vi "Step Update Output.vi"(8 "error in (no error)":errorcluster, 10 "Output in":T1, 11 "Step in":refnum<class "Step.lvclass">) -> (0 "error out":errorcluster, 3 "Step out":refnum<class "Step.lvclass">)   [LabVIEW 2015, in "OutputUI.lvclass"]
uses:
  OutputUI.lvclass
  Step.lvclass
  Step/STEP_OUTPUT.ctl
  Step/OUTPUT_DATA_TYPE.ctl
  OUTPUT_CHECK_TYPE.ctl
  Step/OUTPUT_VALUE_TYPE.ctl
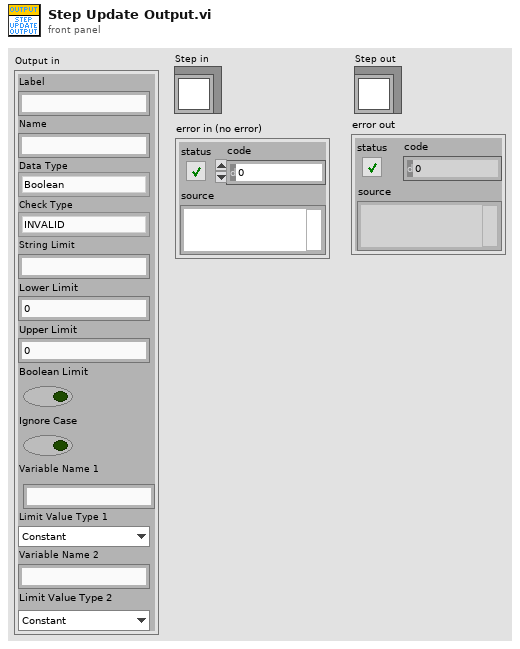
[diagram p1: front panel]
types:
  T1 = typedef "Step.lvclass/STEP_OUTPUT.ctl" = cluster{"Label":string, "Name":string, "Data Type":T2, "Check Type":T3, "String Limit":string, "Lower Limit":dbl, "Upper Limit":dbl, "Boolean Limit":bool, "Ignore Case":bool, "Variable Name 1":string, "Limit Value Type 1":T4, "Variable Name 2":string, "Limit Value Type 2":T4}
  T2 = typedef "Step.lvclass/OUTPUT_DATA_TYPE.ctl" = enum16{"Boolean", "String", "Numeric", "Other"}
  T3 = typedef "Step.lvclass/OUTPUT_CHECK_TYPE.ctl" = enum16{"INVALID", "DO_NOT_CHECK", "RECORD", "VARIABLE", "EQUAL", "NOT_EQUAL", "STR_CONTAINS", "STR_START_WITH", "STR_END_WITH", "STR_REGEX_MATCH", "NUM_GT", "NUM_LT", "NUM_GE", "NUM_LE", "NUM_RANGE", "NUM_RANGE_BDY"}
  T4 = typedef "Step.lvclass/OUTPUT_VALUE_TYPE.ctl" = enum16{"Constant", "Variable"}
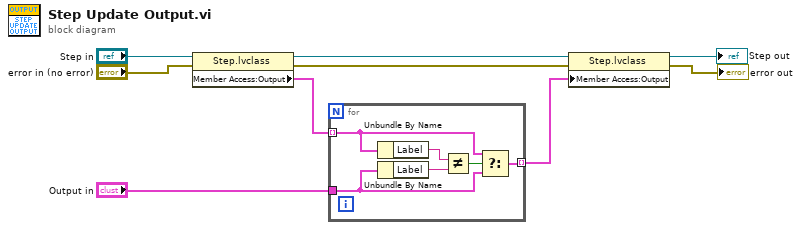
[diagram p0: block diagram]
diagram:
  n1 = property class="Step.lvclass"(reference="Step in", error in="error in (no error)") -> (reference out=w5:refnum<class "Step.lvclass">, error out=w4:errorcluster, "Member Access:Output"=w7:T1[])
  n2 = for {
    tunnel: w7 -> [w12] mode=indexing
    tunnel: "Output in" -> [w11]
    tunnel: [w10] -> w1 mode=indexing
    n3 = Unbundle By Name(w12) -> ("Label"=w14:string)
    n4 = Unbundle By Name(w11) -> ("Label"=w15:string)
    n5 = Not Equal?(x=w14, y=w15) -> (x != y?=w13:bool)
    n6 = Select(t=w12, s=w13, f=w11) -> (s? t:f=w10:T1)
  }
  n7 = property class="Step.lvclass"(reference=w5, error in=w4, "Member Access:Output"=w1) -> (reference out=→"Step out":refnum<class "Step.lvclass">, error out=→"error out":errorcluster)
